vi "Move to (SubVI).vi"(7 "Instrument":T1={"limit"={"Field limit"=0.0, "Field rate limit"=0.0, "Temp limit"=0.0, "Temp low limit"=0.0, "Temp rate limit "=0.0}, "genarl"={"行数"=refnum, "编辑列表框？"=refnum, "列表框"=refnum, "camg 振荡状态"=refnum, "Aborting"=refnum, "数据文件"=refnum, "warning"=refnum, "vi路径"="", "Instrument Type"=enum."PPMS-Rotate"}, "cmag"={"TM620"="TCPIP0::192.168.1.5::4266::SOCKET", "M24C Resource"="GPIB0::24::INSTR", "4G supply"="", "Temp Status 24C"=refnum, "Temp"=refnum, "9T信号"=refnum, "4g supply status"=refnum, "in-plane"="", "out-plane"="", "in-plane signal"=FALSE, "out-plane signal"=FALSE, "in plane 信号"=refnum, "pzt volt"=refnum, "camg Rate"=refnum}, "lengtou2"={"750 visa"="", "750 rotate"="", "semaphore 340"=refnum, "semaphore 750"=refnum, "750 field status"=refnum, "Input (0:A) 340"=0, "340 Resource"="GPIB0::14::INSTR", "340 Status"=refnum, "Input (0:B) 340"=1, "Loop (0: 1)"=0, "Loop (1: 1)"=0, "TCP master instance"=refnum}, "lengtou"={"TCP master instance"=refnum, "335 Status"=refnum, "335 Resource "="GPIB0::24::INSTR", "Input (0:A) 335"=0, "Input (0:B) 335"=1, "Heater Output (1:1) 335"=1, "semaphore 335"=refnum}, "325 for test"={"quantum design"=refnum, "semaphore 325"=refnum, "325 Resource "="GPIB0::13::INSTR", "Input (0:A) 325"=0, "Heater Output (1:1) 325"=1, "325 Status"=refnum}} {"325 for test"."Heater Output (1:1) 325" items=["1"=1, "2"=2]; "325 for test"."Input (0:A) 325" items=["A", "B"]; "lengtou"."Heater Output (1:1) 335" items=["1"=1, "2"=2]; "lengtou"."Input (0:B) 335" items=["A", "B"]; "lengtou"."Input (0:A) 335" items=["A", "B"]; "lengtou2"."Loop (1: 1)" items=["1", "2"]; "lengtou2"."Loop (0: 1)" items=["1", "2"]; "lengtou2"."Input (0:B) 340" items=["A", "B", "C", "D"]; "lengtou2"."Input (0:A) 340" items=["A", "B", "C", "D"]}, 10 "字符串":string) -> (0 "错误输出":errorcluster)   [LabVIEW 2019, in "Take Seq.lvlib"]
uses:
  Take Seq.lvlib
  ctl/Instrument.ctl
  <vilib>/NI/Modbus Library/API/Master/Modbus Master.lvclass
  ctl/limit.ctl
  ctl/warning.ctl
  ctl/Instrument Type.ctl
  ctl/335 state.ctl
  ctl/9T mag field stauts.ctl
  C:/Users/fuyang/Desktop/postdoctor/labview/labview-measure/lib/QDInstrument.dll
  lib/QDInstrument.dll
  ctl/set type.ctl
  User lib.lvlib
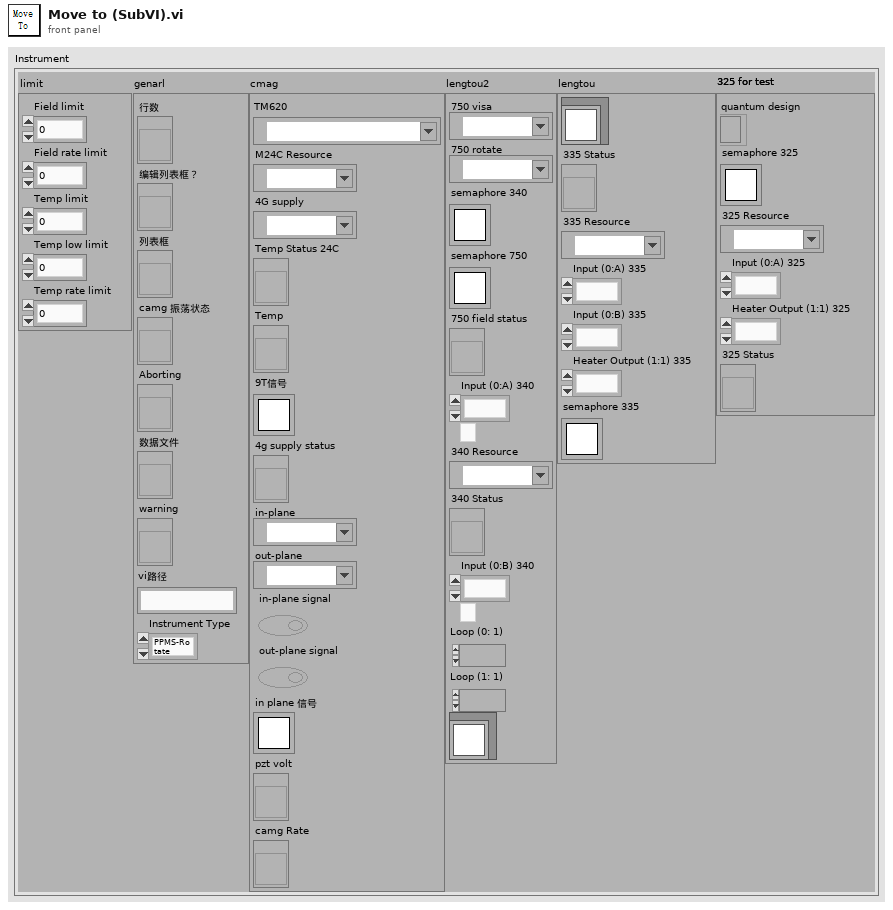
[diagram p1: front panel]
types:
  T1 = typedef "Instrument.ctl" = cluster{"limit":T2, "genarl":cluster{"行数":refnum<vi>, "编辑列表框？":refnum<vi>, "列表框":refnum<vi>, "camg 振荡状态":refnum<vi>, "Aborting":refnum<vi>, "数据文件":refnum<vi>, "warning":refnum<vi>, "vi路径":string, "Instrument Type":T3}, "cmag":cluster{"TM620":refnum<visa-resource-name>, "M24C Resource":refnum<visa-resource-name>, "4G supply":refnum<visa-resource-name>, "Temp Status 24C":refnum<vi>, "Temp":refnum<vi>, "9T信号":T4, "4g supply status":refnum<vi>, "in-plane":refnum<visa-resource-name>, "out-plane":refnum<visa-resource-name>, "in-plane signal":bool, "out-plane signal":bool, "in plane 信号":T4, "pzt volt":refnum<vi>, "camg Rate":refnum<vi>}, "lengtou2":cluster{"750 visa":refnum<visa-resource-name>, "750 rotate":refnum<visa-resource-name>, "semaphore 340":T4, "semaphore 750":T4, "750 field status":refnum<vi>, "Input (0:A) 340":u16, "340 Resource":refnum<visa-resource-name>, "340 Status":refnum<vi>, "Input (0:B) 340":u16, "Loop (0: 1)":u16, "Loop (1: 1)":u16, "TCP master instance":refnum<class "Modbus Master.lvclass">}, "lengtou":cluster{"TCP master instance":refnum<class "Modbus Master.lvclass">, "335 Status":refnum<vi>, "335 Resource ":refnum<visa-resource-name>, "Input (0:A) 335":u16, "Input (0:B) 335":u16, "Heater Output (1:1) 335":u16, "semaphore 335":T4}, "325 for test":cluster{"quantum design":refnum<k24>, "semaphore 325":T4, "325 Resource ":refnum<visa-resource-name>, "Input (0:A) 325":u16, "Heater Output (1:1) 325":u16, "325 Status":refnum<vi>}}
  T2 = typedef "limit.ctl" = cluster{"Field limit":dbl, "Field rate limit":dbl, "Temp limit":dbl, "Temp low limit":dbl, "Temp rate limit ":dbl}
  T3 = typedef "Instrument Type.ctl" = enum16{"PPMS", "VersaLab", "DynaCool", "SVSM", "PPMS-Rotate", "Lakeshore335", "2T cmag", "9T mag old", "9T cmag", "9T cmag DAC", "9T cmag rotate", "test"}
  T4 = typedef "Semaphore RefNum" = refnum<k1>
  T5 = typedef "set type.ctl" = enum16{"temp", "field", "position", "gating", "current", "PZT", "StrainCell", "time"}
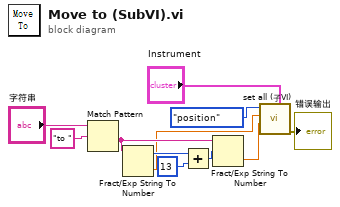
[diagram p0: block diagram]
diagram:
  n1 = Match Pattern(string="字符串", regular expression="to " ("正则表达式")) -> (after substring=w10:string)  [unwired: 1 in, 3 out]
  n2 = Fract/Exp String To Number(string=w10) -> (offset past number=w8:i32, number=w5:dbl)  [unwired: 3 in]
  n3 = Add(x=w8, y=13) -> (x+y=w11:i32)
  n4 = Fract/Exp String To Number(string=w10, offset=w11) -> (number=w4:dbl)  [unwired: 2 in, 1 out]
  n5 = call "set all (子VI).vi"("Instrument"="Instrument", "Rate/speed"=w4, "Target"=w5, "类型"=set_type."position") -> ("error out"=→"错误输出":errorcluster)  [unwired: 7 in]
